vi "Jogo da Velha.vi"(8 "2 Jogadores?":bool=TRUE, 9 "NívelDificuldade":u32, 10 "Jogador 2":string="Jogador 2", 11 "Jogador 1":string="Jogador 1") -> (2 "JogarNovamente?":bool)   [LabVIEW 2011]
doc: "VI responsável por gerenciar o Jogo da Velha, ou seja, a vez de cada jogador, as jogadas feitas e etc."
uses:
  TypeDef/EnumJogadores.ctl
  <vilib>/Utility/sysdir.llb/System Directory Type.ctl
panel:
  in  "JogarNovamente":bool
  out "2x3":string
  in  "stop":bool
  out "Quem joga":string
  out "1x1":string
  out "1x2":string
  out "1x3":string
  out "2x1":string
  out "2x2":string
  out "3x1":string
  out "3x2":string
  out "3x3":string
  # "Jogo da Velha"
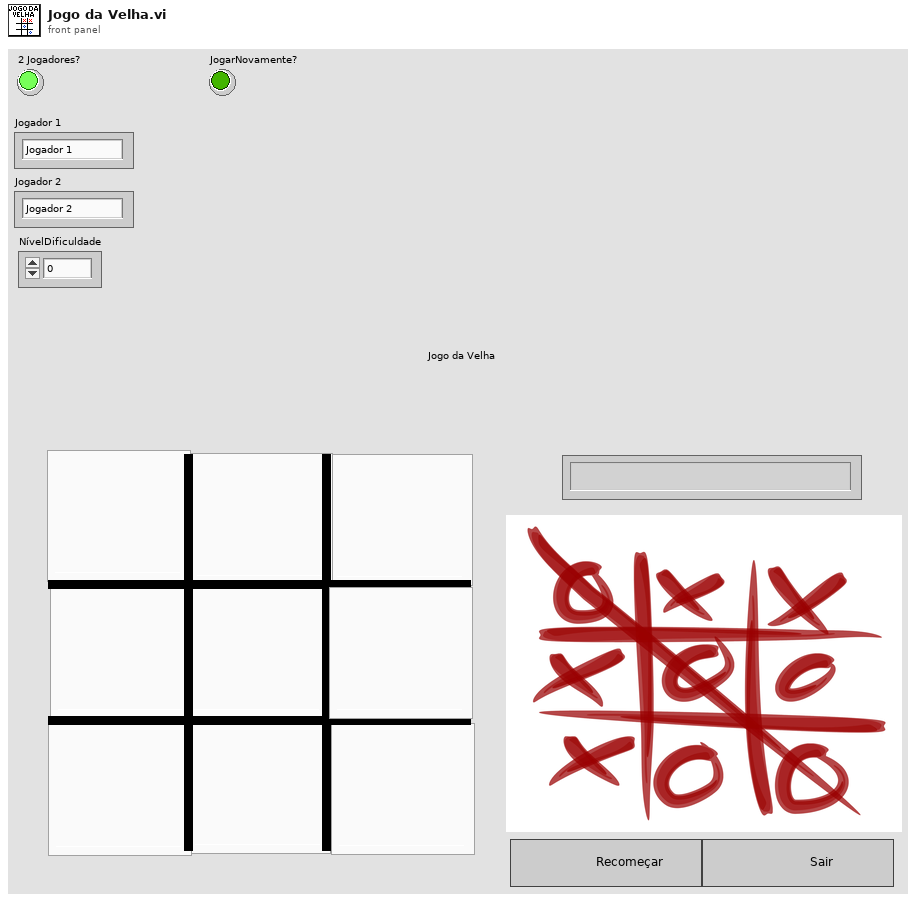
[diagram p1: front panel]
types:
  T1 = typedef "System Directory Type.ctl" = i32
  T2 = enum16{"open", "replace", "create", "open or create", "replace or create", "replace or create with confirmation"}
  T3 = typedef "EnumJogadores.ctl" = enum16{"Jogador 1", "Jogador 2"}
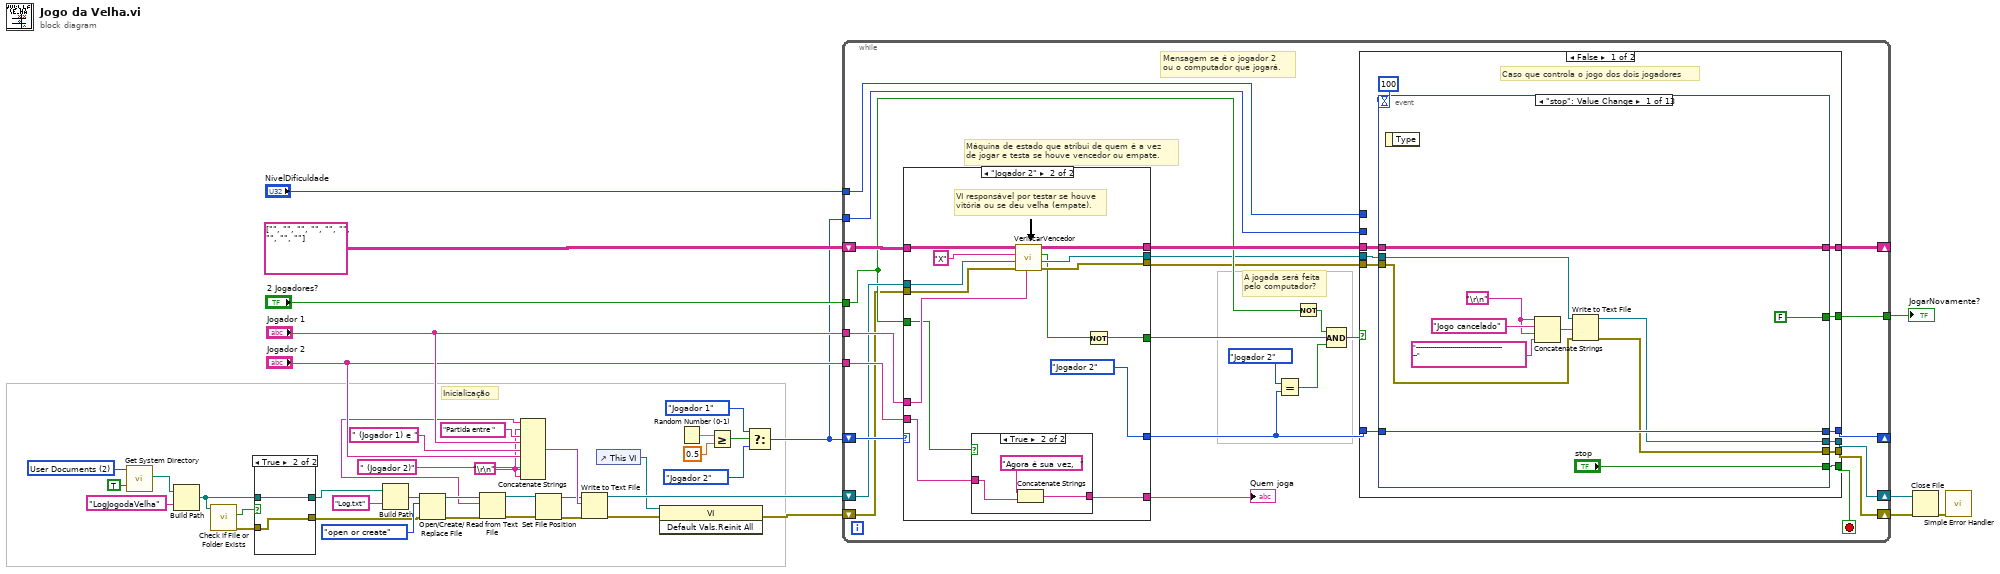
[diagram p0: block diagram]
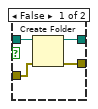
[diagram p2: hidden frame]
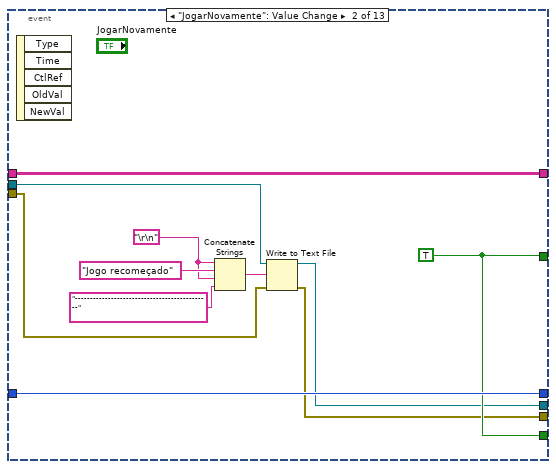
[diagram p3: hidden frame]
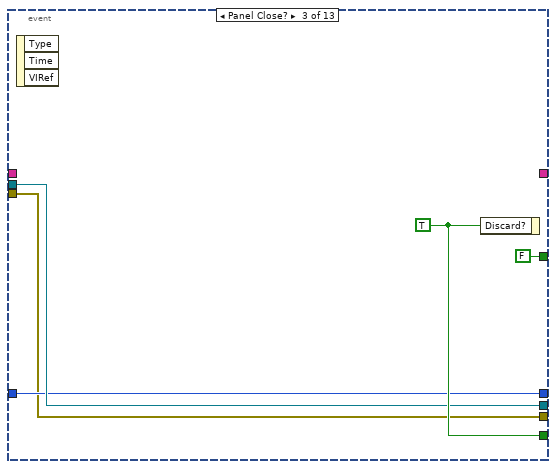
[diagram p4: hidden frame]
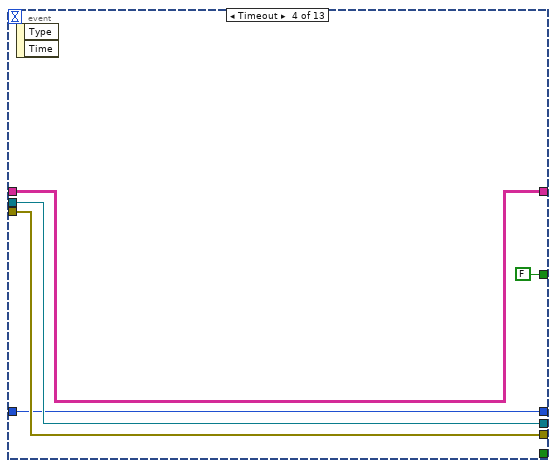
[diagram p5: hidden frame]
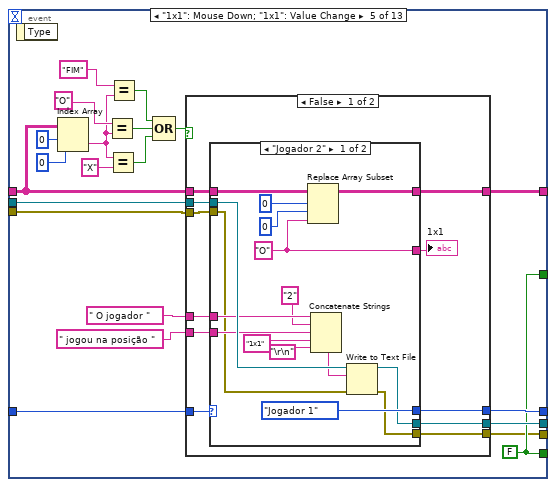
[diagram p6: hidden frame]
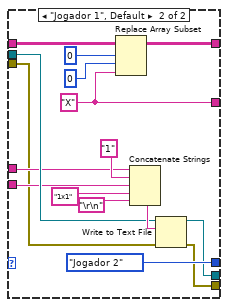
[diagram p7: hidden frame]
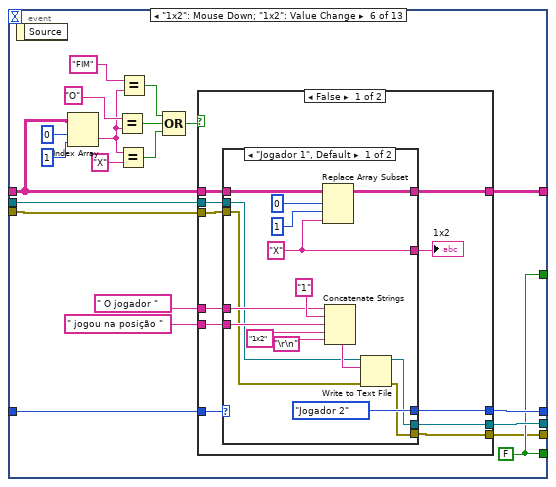
[diagram p9: hidden frame]
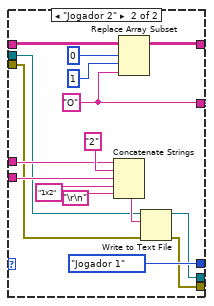
[diagram p10: hidden frame]
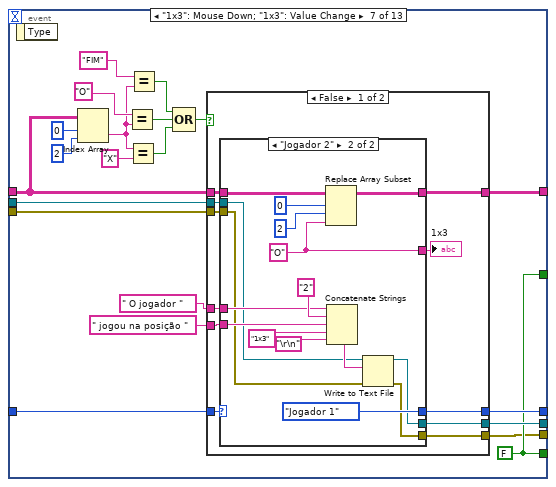
[diagram p12: hidden frame]
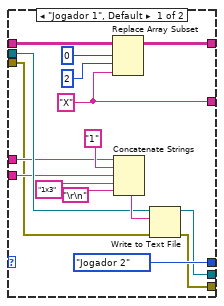
[diagram p13: hidden frame]
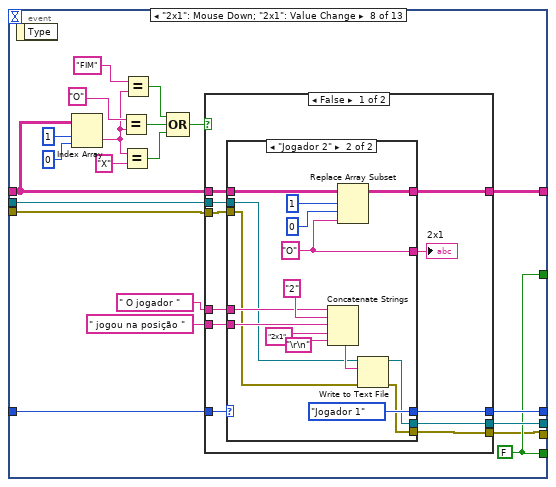
[diagram p15: hidden frame]
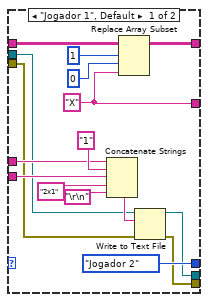
[diagram p16: hidden frame]
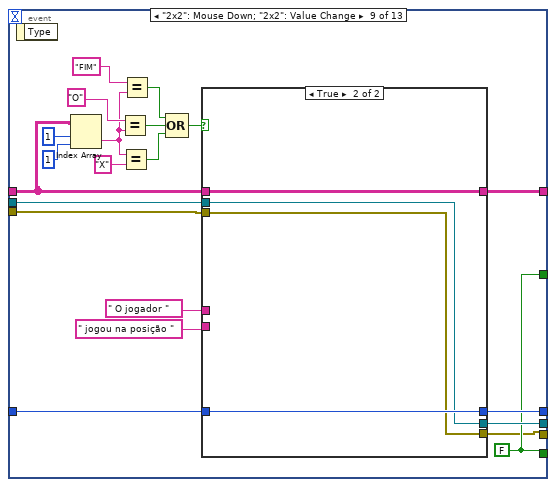
[diagram p18: hidden frame]
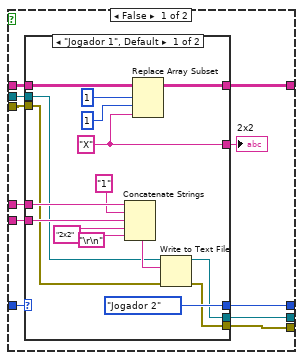
[diagram p19: hidden frame]
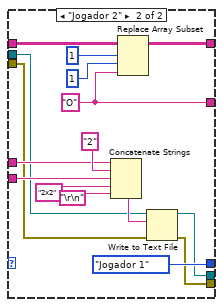
[diagram p20: hidden frame]
diagram:
  w15 = T1 2 items=["User Home"=0, "User Desktop"=1, "User Documents"=2, "User Application Data"=3, "User Preferences"=4, "User Temporary"=5, "Public Documents"=6, "Public Application Data"=7, "Public Preferences"=8, "Public Cache"=13, "System Core Libraries"=9, "System Installed Libraries"=10, "Application Files"=11, "Boot Volume Root"=12] ("system directory type")
  w19 = "\r\n"
  # "Inicialização"
  n1 = call <vilib>:"Get System Directory.vi"("create directory if not found? (F)"=TRUE, "system directory type"=w15) -> ("system directory"=w10:path)  [unwired: 9 in]
  n2 = Build Path(base path=w10, name or relative path="LogJogodaVelha") -> (appended path=w3:path)
  n3 = call <vilib>:"Check if File or Folder Exists.vi"("path"=w3) -> ("error out"=w2:errorcluster, "file or folder exists?"=w1:bool)  [unwired: 8 in, 1 out]
  n4 = case shown="True" w1 {
    tunnel: [w47 w49] -> w8
    tunnel: [w46 w48] -> w7
    tunnel: w3 -> [w45 w49]
    tunnel: w2 -> [w44 w48]
    frame False {
      n5 = Create Folder(path (use dialog)=w45, error in=w44) -> (created path=w47:path, error out=w46:errorcluster)  [unwired: 1 in, 1 out]
    }
    frame True {
    }
  }
  n6 = Build Path(base path=w8, name or relative path="Log.txt") -> (appended path=w13:path)
  n7 = Open/Create/Replace File(file path (use dialog)=w13, error in=w7, operation (0:open)=T2."open or create") -> (refnum out=w27:refnum<file>, error out=w26:errorcluster)  [unwired: 3 in, 1 out]
  n8 = Read from Text File(file (use dialog)=w27, error in=w26) -> (refnum out=w24:refnum<file>, text=w25:string, error out=w22:errorcluster)  [unwired: 2 in, 1 out]
  n9 = Concatenate Strings(w25, w19, "Partida entre " ("string"), "Jogador 1", " (Jogador 1) e " ("string"), "Jogador 2", " (Jogador 2)" ("string"), w19, w19) -> (w31:string)
  n10 = Set File Position(refnum=w24, error in=w22) -> (refnum out=w23:refnum<file>, error out=w21:errorcluster)  [unwired: 2 in]
  n11 = Write to Text File(file (use dialog)=w23, text=w31, error in=w21) -> (refnum out=w29:refnum<file>, error out=w5:errorcluster)  [unwired: 1 in, 1 out]
  n12 = control-ref of="This VI"() -> (w6:refnum<vi>)
  n13 = invoke class="VI" method="Default Vals.Reinit All"(reference=w6, error in=w5) -> (error out=w4:errorcluster)  [unwired: 1 in, 2 out]
  n14 = Random Number (0-1)() -> (number: 0 to 1=w37:dbl)
  n15 = Greater Or Equal?(x=w37, y=0.5) -> (x >= y?=w39:bool)
  n16 = Select(t=EnumJogadores."Jogador 1" ("Enum"), s=w39, f=EnumJogadores."Jogador 2" ("Enum")) -> (s? t:f=w20:T3)
  n17 = while {
    tunnel: "Jogador 2" -> [w70]
    tunnel: "Jogador 1" -> [w71]
    tunnel: "2 Jogadores?" -> [w59]
    shift-right: [w74] -> _
    shift-left: string[][] [["", "", ""], ["", "", ""], ["", "", ""]] ("ArrayJogoVelha") -> [w63]
    shift-right: [w72] -> _
    shift-left: w20 -> [w73]
    tunnel: [w62] -> w36
    shift-right: [w58] -> w28
    shift-left: w29 -> [w60]
    tunnel: w20 -> [w57]
    tunnel: "NívelDificuldade" -> [w51]
    shift-right: [w50] -> w11
    shift-left: w4 -> [w54]
    stop <- w68 stop-if-true
    # "Mensagem se é o jogador 2\nou o computador que jogará."
    # "Máquina de estado que atribui de quem é a vez \nde jogar e testa se houve vencedor ou empate."
    # "A jogada será feita\npelo computador?"
    n18 = case shown="\"Jogador 2\"" w73 {
      tunnel: [EnumJogadores."Jogador 1" ("Enum") EnumJogadores."Jogador 2" ("Enum")] -> w66
      tunnel: w71 -> [w783 w791]
      tunnel: w70 -> [w779 w797]
      tunnel: [w785 w800] -> w69
      tunnel: w59 -> [_ w787]
      tunnel: w63 -> [w784 w798]
      tunnel: [w782 w796] -> w61
      tunnel: w60 -> [w777 w789]
      tunnel: [w780 w794] -> w55
      tunnel: w54 -> [w778 w790]
      tunnel: [w776 w793] -> w53
      tunnel: [w775 w792] -> w52
      frame "Jogador 1" {
        # "VI responsável por testar se houve\nvitória ou se deu velha (empate)."
        n19 = call "VerificarVencedor.vi"("Nome do Jogador"=w779, "error in (no error)"=w778, "refnum in"=w777, "CaracterComparacao"="O", "ArrayEntrada"=w784) -> ("error out"=w775:errorcluster, "refnum out"=w776:refnum<file>, "VenceuOuEmpatou"=w774:bool, "ArraySaida"=w782:string[][])  [unwired: 3 in]
        n20 = Concatenate Strings("Agora é sua vez,  " ("string"), w783) -> (w785:string)
        n21 = Not(x=w774) -> (.not. x?=w780:bool)
      }
      frame "Jogador 2" {
        # "VI responsável por testar se houve\nvitória ou se deu velha (empate)."
        n22 = case shown="True" w787 {
          tunnel: w797 -> [_ w802]
          tunnel: ["Agora é a vez do computador" w803] -> w800
          frame False {
          }
          frame True {
            n23 = Concatenate Strings("Agora é sua vez,  " ("string"), w802) -> (w803:string)
          }
        }
        n24 = call "VerificarVencedor.vi"("Nome do Jogador"=w791, "error in (no error)"=w790, "refnum in"=w789, "CaracterComparacao"="X", "ArrayEntrada"=w798) -> ("error out"=w792:errorcluster, "refnum out"=w793:refnum<file>, "VenceuOuEmpatou"=w788:bool, "ArraySaida"=w796:string[][])  [unwired: 3 in]
        n25 = Not(x=w788) -> (.not. x?=w794:bool)
      }
    }
    "Quem joga" <- w69
    n26 = Equal?(x=EnumJogadores."Jogador 2" ("Enum"), y=w66) -> (x = y?=w56:bool)
    n27 = Not(x=w59) -> (.not. x?=w64:bool)
    n28 = Compound Arithmetic op=AND(w64, w55, w56) -> (w67:bool)
    n29 = case shown="False" w67 {
      tunnel: w61 -> [w85 w732]
      tunnel: [w84 w739] -> w74
      tunnel: w66 -> [w83 _]
      tunnel: [w82 EnumJogadores."Jogador 1" ("Enum")] -> w72
      tunnel: [w81 FALSE ("stop")] -> w68
      tunnel: [w80 FALSE] -> w62
      tunnel: w53 -> [w78 w738]
      tunnel: [w79 w737] -> w58
      tunnel: w57 -> [_ w742]
      tunnel: w52 -> [w77 w734]
      tunnel: [w76 w736] -> w50
      tunnel: w51 -> [_ w735]
      frame False {
        # "Caso que controla o jogo dos dois jogadores"
        n30 = event shown="[0] \"stop\": Value Change" {
          selector: _ -> [_ _ _ _ _ _ _ _ _ _ _ _ _]
          dyn-events: _ -> [_ _ _ _ _ _ _ _ _ _ _ _ _]
          timeout: 100 -> [_ _ _ _ _ _ _ _ _ _ _ _ _]
          tunnel: w85 -> [w96 w108 _ w114 w138 w195 w264 w331 w400 w467 w536 w604 w672]
          tunnel: [w96 w108 _ w114 w139 w207 w275 w343 w411 w479 w547 w615 w683] -> w84
          tunnel: w83 -> [w95 w107 w111 w115 w135 w206 w274 w342 w410 w478 w546 w614 w682]
          tunnel: [w95 w107 w111 w115 w134 w205 w273 w341 w409 w477 w545 w613 w681] -> w82
          tunnel: ["stop" w106 w113 _ w121 w190 w257 w325 w393 w461 w529 w597 w665] -> w81
          tunnel: [FALSE w106 FALSE FALSE w121 w190 w257 w325 w393 w461 w529 w597 w665] -> w80
          tunnel: w78 -> [w90 w102 w112 w118 w125 w189 w261 w329 w397 w465 w533 w601 w669]
          tunnel: [w89 w101 w112 w118 w124 w193 w260 w328 w396 w464 w532 w600 w668] -> w79
          tunnel: w77 -> [w87 w99 w110 w117 w120 w188 w256 w324 w392 w460 w528 w596 w664]
          tunnel: [w86 w98 w110 w117 w119 w187 w255 w323 w391 w459 w527 w595 w663] -> w76
          event "stop": Value Change {
            w91 = "\r\n"
            n31 = event-data() -> ()  [unwired: 1 in, 1 out]
            n32 = Concatenate Strings(w91, "Jogo cancelado" ("string"), w91, "---------------------------------------------" ("string")) -> (w93:string)
            n33 = Write to Text File(file (use dialog)=w90, text=w93, error in=w87) -> (refnum out=w89:refnum<file>, error out=w86:errorcluster)  [unwired: 1 in, 1 out]
          }
          event "JogarNovamente": Value Change {
            w103 = "\r\n"
            w106 = TRUE
            n34 = event-data() -> ()  [unwired: 1 in, 5 out]
            n35 = Concatenate Strings(w103, "Jogo recomeçado" ("string"), w103, "---------------------------------------------" ("string")) -> (w105:string)
            n36 = Write to Text File(file (use dialog)=w102, text=w105, error in=w99) -> (refnum out=w101:refnum<file>, error out=w98:errorcluster)  [unwired: 1 in, 1 out]
          }
          event Panel Close? {
            w113 = TRUE ("Discard?")
            n37 = event-data() -> ()  [unwired: 1 in, 3 out]
            n38 = event-data("Discard?"=w113) -> ()  [unwired: 1 in, 1 out]
          }
          event Timeout {
            n39 = event-data() -> ()  [unwired: 1 in, 2 out]
          }
          event "1x1": Mouse Down; "1x1": Value Change {
            w121 = FALSE
            n40 = event-data() -> ()  [unwired: 1 in, 1 out]
            n41 = Index Array(array=w138, index (row)=0, index (col)=0 ("disabled index (col)")) -> (element=w128:string)
            n42 = Equal?(x="O", y=w128) -> (x = y?=w130:bool)
            n43 = Equal?(x=w128, y="X") -> (x = y?=w131:bool)
            n44 = Equal?(x="FIM", y=w128) -> (x = y?=w126:bool)
            n45 = Compound Arithmetic op=OR(w126, w130, w131) -> (w132:bool)
            n46 = case shown="False" w132 {
              tunnel: w138 -> [w150 w186]
              tunnel: [w149 w186] -> w139
              tunnel: w135 -> [w147 w183]
              tunnel: [w146 w183] -> w134
              tunnel: w125 -> [w145 w185]
              tunnel: [w144 w185] -> w124
              tunnel: " O jogador " ("string") -> [w143 _]
              tunnel: " jogou na posição " ("string") -> [w142 _]
              tunnel: w120 -> [w141 w184]
              tunnel: [w140 w184] -> w119
              frame False {
                n47 = case shown="\"Jogador 2\"" w147 {
                  tunnel: w150 -> [w164 w180]
                  tunnel: [w163 w179] -> w149
                  tunnel: [w162 w178] -> w148
                  tunnel: [EnumJogadores."Jogador 1" ("Enum") EnumJogadores."Jogador 2" ("Enum")] -> w146
                  tunnel: w145 -> [w159 w172]
                  tunnel: [w160 w169] -> w144
                  tunnel: w143 -> [w157 w171]
                  tunnel: w142 -> [w156 w170]
                  tunnel: w141 -> [w152 w168]
                  tunnel: [w151 w167] -> w140
                  frame "Jogador 2" {
                    w162 = "O" ("new element/subarray")
                    n48 = Replace Array Subset(array=w164, new element=w162, index (row)=0, index (col)=0 ("disabled index (col)")) -> (w163:string[][])
                    n49 = Concatenate Strings(w157, "2" ("string"), w156, "1x1" ("string"), "\r\n") -> (w158:string)
                    n50 = Write to Text File(file (use dialog)=w159, text=w158, error in=w152) -> (refnum out=w160:refnum<file>, error out=w151:errorcluster)  [unwired: 1 in, 1 out]
                  }
                  frame "Jogador 1", Default {
                    w178 = "X" ("new element/subarray")
                    n51 = Replace Array Subset(array=w180, new element=w178, index (row)=0, index (col)=0 ("disabled index (col)")) -> (w179:string[][])
                    n52 = Concatenate Strings(w171, "1" ("string"), w170, "1x1" ("string"), "\r\n") -> (w173:string)
                    n53 = Write to Text File(file (use dialog)=w172, text=w173, error in=w168) -> (refnum out=w169:refnum<file>, error out=w167:errorcluster)  [unwired: 1 in, 1 out]
                  }
                }
                "1x1" <- w148
              }
              frame True {
              }
            }
          }
          event "1x2": Mouse Down; "1x2": Value Change {
            w190 = FALSE
            n54 = event-data() -> ()  [unwired: 1 in, 1 out]
            n55 = Index Array(array=w195, index (row)=0, index (col)=1 ("disabled index (col)")) -> (element=w200:string)
            n56 = Equal?(x="O", y=w200) -> (x = y?=w202:bool)
            n57 = Equal?(x=w200, y="X") -> (x = y?=w203:bool)
            n58 = Equal?(x="FIM", y=w200) -> (x = y?=w198:bool)
            n59 = Compound Arithmetic op=OR(w198, w202, w203) -> (w194:bool)
            n60 = case shown="False" w194 {
              tunnel: w195 -> [w218 w254]
              tunnel: [w217 w254] -> w207
              tunnel: w206 -> [w215 w253]
              tunnel: [w214 w253] -> w205
              tunnel: w189 -> [w213 w252]
              tunnel: [w212 w252] -> w193
              tunnel: " O jogador " ("string") -> [w211 _]
              tunnel: " jogou na posição " ("string") -> [w210 _]
              tunnel: w188 -> [w209 w251]
              tunnel: [w208 w251] -> w187
              frame False {
                n61 = case shown="\"Jogador 1\", Default" w215 {
                  tunnel: w218 -> [w234 w248]
                  tunnel: [w233 w247] -> w217
                  tunnel: [w230 w246] -> w216
                  tunnel: [EnumJogadores."Jogador 2" ("Enum") EnumJogadores."Jogador 1" ("Enum")] -> w214
                  tunnel: w213 -> [w221 w237]
                  tunnel: [w222 w238] -> w212
                  tunnel: w211 -> [w224 w240]
                  tunnel: w210 -> [w223 w239]
                  tunnel: w209 -> [w220 w236]
                  tunnel: [w219 w235] -> w208
                  frame "Jogador 1", Default {
                    w230 = "X" ("new element/subarray")
                    n62 = Replace Array Subset(array=w234, new element=w230, index (row)=0, index (col)=1 ("disabled index (col)")) -> (w233:string[][])
                    n63 = Concatenate Strings(w224, "1" ("string"), w223, "1x2" ("string"), "\r\n") -> (w225:string)
                    n64 = Write to Text File(file (use dialog)=w221, text=w225, error in=w220) -> (refnum out=w222:refnum<file>, error out=w219:errorcluster)  [unwired: 1 in, 1 out]
                  }
                  frame "Jogador 2" {
                    w246 = "O" ("new element/subarray")
                    n65 = Concatenate Strings(w240, "2" ("string"), w239, "1x2" ("string"), "\r\n") -> (w241:string)
                    n66 = Replace Array Subset(array=w248, new element=w246, index (row)=0, index (col)=1 ("disabled index (col)")) -> (w247:string[][])
                    n67 = Write to Text File(file (use dialog)=w237, text=w241, error in=w236) -> (refnum out=w238:refnum<file>, error out=w235:errorcluster)  [unwired: 1 in, 1 out]
                  }
                }
                "1x2" <- w216
              }
              frame True {
              }
            }
          }
          event "1x3": Mouse Down; "1x3": Value Change {
            w257 = FALSE
            n68 = event-data() -> ()  [unwired: 1 in, 1 out]
            n69 = Index Array(array=w264, index (row)=0, index (col)=2 ("disabled index (col)")) -> (element=w268:string)
            n70 = Equal?(x="O", y=w268) -> (x = y?=w270:bool)
            n71 = Equal?(x=w268, y="X") -> (x = y?=w271:bool)
            n72 = Equal?(x="FIM", y=w268) -> (x = y?=w266:bool)
            n73 = Compound Arithmetic op=OR(w266, w270, w271) -> (w263:bool)
            n74 = case shown="False" w263 {
              tunnel: w264 -> [w286 w322]
              tunnel: [w285 w322] -> w275
              tunnel: w274 -> [w283 w321]
              tunnel: [w282 w321] -> w273
              tunnel: w261 -> [w281 w320]
              tunnel: [w280 w320] -> w260
              tunnel: " jogou na posição " ("string") -> [w279 _]
              tunnel: " O jogador " ("string") -> [w278 _]
              tunnel: w256 -> [w277 w319]
              tunnel: [w276 w319] -> w255
              frame False {
                n75 = case shown="\"Jogador 2\"" w283 {
                  tunnel: w286 -> [w300 w316]
                  tunnel: [w299 w315] -> w285
                  tunnel: [w298 w314] -> w284
                  tunnel: [EnumJogadores."Jogador 2" ("Enum") EnumJogadores."Jogador 1" ("Enum")] -> w282
                  tunnel: w281 -> [w291 w305]
                  tunnel: [w292 w306] -> w280
                  tunnel: w279 -> [w289 w307]
                  tunnel: w278 -> [w290 w308]
                  tunnel: w277 -> [w288 w304]
                  tunnel: [w287 w303] -> w276
                  frame "Jogador 1", Default {
                    w298 = "X" ("new element/subarray")
                    n76 = Replace Array Subset(array=w300, new element=w298, index (row)=0, index (col)=2 ("disabled index (col)")) -> (w299:string[][])
                    n77 = Concatenate Strings(w290, "1" ("string"), w289, "1x3" ("string"), "\r\n") -> (w296:string)
                    n78 = Write to Text File(file (use dialog)=w291, text=w296, error in=w288) -> (refnum out=w292:refnum<file>, error out=w287:errorcluster)  [unwired: 1 in, 1 out]
                  }
                  frame "Jogador 2" {
                    w314 = "O" ("new element/subarray")
                    n79 = Replace Array Subset(array=w316, new element=w314, index (row)=0, index (col)=2 ("disabled index (col)")) -> (w315:string[][])
                    n80 = Concatenate Strings(w308, "2" ("string"), w307, "1x3" ("string"), "\r\n") -> (w309:string)
                    n81 = Write to Text File(file (use dialog)=w305, text=w309, error in=w304) -> (refnum out=w306:refnum<file>, error out=w303:errorcluster)  [unwired: 1 in, 1 out]
                  }
                }
                "1x3" <- w284
              }
              frame True {
              }
            }
          }
          event "2x1": Mouse Down; "2x1": Value Change {
            w325 = FALSE
            n82 = event-data() -> ()  [unwired: 1 in, 1 out]
            n83 = Index Array(array=w331, index (row)=1, index (col)=0 ("disabled index (col)")) -> (element=w336:string)
            n84 = Equal?(x="O", y=w336) -> (x = y?=w338:bool)
            n85 = Equal?(x=w336, y="X") -> (x = y?=w339:bool)
            n86 = Equal?(x="FIM", y=w336) -> (x = y?=w334:bool)
            n87 = Compound Arithmetic op=OR(w334, w338, w339) -> (w330:bool)
            n88 = case shown="False" w330 {
              tunnel: w331 -> [w354 w390]
              tunnel: [w353 w390] -> w343
              tunnel: w342 -> [w351 w389]
              tunnel: [w350 w389] -> w341
              tunnel: w329 -> [w349 w387]
              tunnel: [w348 w387] -> w328
              tunnel: " O jogador " ("string") -> [w347 _]
              tunnel: " jogou na posição " ("string") -> [w346 _]
              tunnel: w324 -> [w345 w388]
              tunnel: [w344 w388] -> w323
              frame False {
                n89 = case shown="\"Jogador 2\"" w351 {
                  tunnel: w354 -> [w368 w384]
                  tunnel: [w367 w383] -> w353
                  tunnel: [w366 w382] -> w352
                  tunnel: [EnumJogadores."Jogador 2" ("Enum") EnumJogadores."Jogador 1" ("Enum")] -> w350
                  tunnel: w349 -> [w357 w373]
                  tunnel: [w358 w376] -> w348
                  tunnel: w347 -> [w360 w375]
                  tunnel: w346 -> [w359 w374]
                  tunnel: w345 -> [w356 w372]
                  tunnel: [w355 w371] -> w344
                  frame "Jogador 1", Default {
                    w366 = "X" ("new element/subarray")
                    n90 = Concatenate Strings(w360, "1" ("string"), w359, "2x1" ("string"), "\r\n") -> (w361:string)
                    n91 = Replace Array Subset(array=w368, new element=w366, index (row)=1, index (col)=0 ("disabled index (col)")) -> (w367:string[][])
                    n92 = Write to Text File(file (use dialog)=w357, text=w361, error in=w356) -> (refnum out=w358:refnum<file>, error out=w355:errorcluster)  [unwired: 1 in, 1 out]
                  }
                  frame "Jogador 2" {
                    w382 = "O" ("new element/subarray")
                    n93 = Concatenate Strings(w375, "2" ("string"), w374, "2x1" ("string"), "\r\n") -> (w378:string)
                    n94 = Replace Array Subset(array=w384, new element=w382, index (row)=1, index (col)=0 ("disabled index (col)")) -> (w383:string[][])
                    n95 = Write to Text File(file (use dialog)=w373, text=w378, error in=w372) -> (refnum out=w376:refnum<file>, error out=w371:errorcluster)  [unwired: 1 in, 1 out]
                  }
                }
                "2x1" <- w352
              }
              frame True {
              }
            }
          }
          event "2x2": Mouse Down; "2x2": Value Change {
            w393 = FALSE
            n96 = event-data() -> ()  [unwired: 1 in, 1 out]
            n97 = Index Array(array=w400, index (row)=1, index (col)=1 ("disabled index (col)")) -> (element=w404:string)
            n98 = Equal?(x="O", y=w404) -> (x = y?=w406:bool)
            n99 = Equal?(x=w404, y="X") -> (x = y?=w407:bool)
            n100 = Equal?(x="FIM", y=w404) -> (x = y?=w402:bool)
            n101 = Compound Arithmetic op=OR(w402, w406, w407) -> (w398:bool)
            n102 = case shown="True" w398 {
              tunnel: w400 -> [w422 w458]
              tunnel: [w421 w458] -> w411
              tunnel: w410 -> [w419 w457]
              tunnel: [w418 w457] -> w409
              tunnel: w397 -> [w417 w456]
              tunnel: [w414 w456] -> w396
              tunnel: " O jogador " ("string") -> [w416 _]
              tunnel: " jogou na posição " ("string") -> [w415 _]
              tunnel: w392 -> [w413 w455]
              tunnel: [w412 w455] -> w391
              frame False {
                n103 = case shown="\"Jogador 1\", Default" w419 {
                  tunnel: w422 -> [w436 w452]
                  tunnel: [w435 w451] -> w421
                  tunnel: [w434 w450] -> w420
                  tunnel: [EnumJogadores."Jogador 2" ("Enum") EnumJogadores."Jogador 1" ("Enum")] -> w418
                  tunnel: w417 -> [w425 w441]
                  tunnel: w416 -> [w429 w444]
                  tunnel: w415 -> [w428 w443]
                  tunnel: [w426 w442] -> w414
                  tunnel: w413 -> [w424 w440]
                  tunnel: [w423 w439] -> w412
                  frame "Jogador 1", Default {
                    w434 = "X" ("new element/subarray")
                    n104 = Concatenate Strings(w429, "1" ("string"), w428, "2x2" ("string"), "\r\n") -> (w430:string)
                    n105 = Replace Array Subset(array=w436, new element=w434, index (row)=1, index (col)=1 ("disabled index (col)")) -> (w435:string[][])
                    n106 = Write to Text File(file (use dialog)=w425, text=w430, error in=w424) -> (refnum out=w426:refnum<file>, error out=w423:errorcluster)  [unwired: 1 in, 1 out]
                  }
                  frame "Jogador 2" {
                    w450 = "O" ("new element/subarray")
                    n107 = Concatenate Strings(w444, "2" ("string"), w443, "2x2" ("string"), "\r\n") -> (w446:string)
                    n108 = Replace Array Subset(array=w452, new element=w450, index (row)=1, index (col)=1 ("disabled index (col)")) -> (w451:string[][])
                    n109 = Write to Text File(file (use dialog)=w441, text=w446, error in=w440) -> (refnum out=w442:refnum<file>, error out=w439:errorcluster)  [unwired: 1 in, 1 out]
                  }
                }
                "2x2" <- w420
              }
              frame True {
              }
            }
          }
          event "2x3": Mouse Down; "2x3": Value Change {
            w461 = FALSE
            n110 = event-data() -> ()  [unwired: 1 in, 1 out]
            n111 = Index Array(array=w467, index (row)=1, index (col)=2 ("disabled index (col)")) -> (element=w472:string)
            n112 = Equal?(x="O", y=w472) -> (x = y?=w474:bool)
            n113 = Equal?(x=w472, y="X") -> (x = y?=w475:bool)
            n114 = Equal?(x="FIM", y=w472) -> (x = y?=w470:bool)
            n115 = Compound Arithmetic op=OR(w470, w474, w475) -> (w466:bool)
            n116 = case shown="True" w466 {
              tunnel: w467 -> [w490 w526]
              tunnel: [w489 w526] -> w479
              tunnel: w478 -> [w484 w525]
              tunnel: [w487 w525] -> w477
              tunnel: w465 -> [w486 w524]
              tunnel: [w485 w524] -> w464
              tunnel: " O jogador " ("string") -> [w483 _]
              tunnel: " jogou na posição " ("string") -> [w482 _]
              tunnel: w460 -> [w481 w523]
              tunnel: [w480 w523] -> w459
              frame False {
                n117 = case shown="\"Jogador 2\"" w484 {
                  tunnel: w490 -> [w504 w521]
                  tunnel: [w503 w520] -> w489
                  tunnel: [w502 w518] -> w488
                  tunnel: [EnumJogadores."Jogador 2" ("Enum") EnumJogadores."Jogador 1" ("Enum")] -> w487
                  tunnel: w486 -> [w494 w512]
                  tunnel: [w493 w511] -> w485
                  tunnel: w483 -> [w496 w510]
                  tunnel: w482 -> [w495 w509]
                  tunnel: w481 -> [w492 w508]
                  tunnel: [w491 w507] -> w480
                  frame "Jogador 1", Default {
                    w502 = "X" ("new element/subarray")
                    n118 = Concatenate Strings(w496, "1" ("string"), w495, "2x3" ("string"), "\r\n") -> (w497:string)
                    n119 = Replace Array Subset(array=w504, new element=w502, index (row)=1, index (col)=2 ("disabled index (col)")) -> (w503:string[][])
                    n120 = Write to Text File(file (use dialog)=w494, text=w497, error in=w492) -> (refnum out=w493:refnum<file>, error out=w491:errorcluster)  [unwired: 1 in, 1 out]
                  }
                  frame "Jogador 2" {
                    w518 = "O" ("new element/subarray")
                    n121 = Concatenate Strings(w510, "2" ("string"), w509, "2x3" ("string"), "\r\n") -> (w513:string)
                    n122 = Replace Array Subset(array=w521, new element=w518, index (row)=1, index (col)=2 ("disabled index (col)")) -> (w520:string[][])
                    n123 = Write to Text File(file (use dialog)=w512, text=w513, error in=w508) -> (refnum out=w511:refnum<file>, error out=w507:errorcluster)  [unwired: 1 in, 1 out]
                  }
                }
                "2x3" <- w488
              }
              frame True {
              }
            }
          }
          event "3x1": Mouse Down; "3x1": Value Change {
            w529 = FALSE
            n124 = event-data() -> ()  [unwired: 1 in, 1 out]
            n125 = Index Array(array=w536, index (row)=2, index (col)=0 ("disabled index (col)")) -> (element=w540:string)
            n126 = Equal?(x="O", y=w540) -> (x = y?=w542:bool)
            n127 = Equal?(x=w540, y="X") -> (x = y?=w543:bool)
            n128 = Equal?(x="FIM", y=w540) -> (x = y?=w538:bool)
            n129 = Compound Arithmetic op=OR(w538, w542, w543) -> (w537:bool)
            n130 = case shown="False" w537 {
              tunnel: w536 -> [w558 w594]
              tunnel: [w557 w594] -> w547
              tunnel: w546 -> [w555 w593]
              tunnel: [w554 w593] -> w545
              tunnel: w533 -> [w553 w592]
              tunnel: [w552 w592] -> w532
              tunnel: " O jogador " ("string") -> [w551 _]
              tunnel: " jogou na posição " ("string") -> [w550 _]
              tunnel: w528 -> [w549 w591]
              tunnel: [w548 w591] -> w527
              frame False {
                n131 = case shown="\"Jogador 2\"" w555 {
                  tunnel: w558 -> [w572 w588]
                  tunnel: [w571 w587] -> w557
                  tunnel: [w570 w586] -> w556
                  tunnel: [EnumJogadores."Jogador 2" ("Enum") EnumJogadores."Jogador 1" ("Enum")] -> w554
                  tunnel: w553 -> [w561 w577]
                  tunnel: [w562 w580] -> w552
                  tunnel: w551 -> [w564 w579]
                  tunnel: w550 -> [w563 w578]
                  tunnel: w549 -> [w560 w576]
                  tunnel: [w559 w575] -> w548
                  frame "Jogador 1", Default {
                    w570 = "X" ("new element/subarray")
                    n132 = Concatenate Strings(w564, "1" ("string"), w563, "3x1" ("string"), "\r\n") -> (w565:string)
                    n133 = Replace Array Subset(array=w572, new element=w570, index (row)=2, index (col)=0 ("disabled index (col)")) -> (w571:string[][])
                    n134 = Write to Text File(file (use dialog)=w561, text=w565, error in=w560) -> (refnum out=w562:refnum<file>, error out=w559:errorcluster)  [unwired: 1 in, 1 out]
                  }
                  frame "Jogador 2" {
                    w586 = "O" ("new element/subarray")
                    n135 = Concatenate Strings(w579, "2" ("string"), w578, "3x1" ("string"), "\r\n") -> (w581:string)
                    n136 = Replace Array Subset(array=w588, new element=w586, index (row)=2, index (col)=0 ("disabled index (col)")) -> (w587:string[][])
                    n137 = Write to Text File(file (use dialog)=w577, text=w581, error in=w576) -> (refnum out=w580:refnum<file>, error out=w575:errorcluster)  [unwired: 1 in, 1 out]
                  }
                }
                "3x1" <- w556
              }
              frame True {
              }
            }
          }
          event "3x2": Mouse Down; "3x2": Value Change {
            w597 = FALSE
            n138 = event-data() -> ()  [unwired: 1 in, 1 out]
            n139 = Index Array(array=w604, index (row)=2, index (col)=1 ("disabled index (col)")) -> (element=w608:string)
            n140 = Equal?(x="O", y=w608) -> (x = y?=w610:bool)
            n141 = Equal?(x=w608, y="X") -> (x = y?=w611:bool)
            n142 = Equal?(x="FIM", y=w608) -> (x = y?=w606:bool)
            n143 = Compound Arithmetic op=OR(w606, w610, w611) -> (w602:bool)
            n144 = case shown="False" w602 {
              tunnel: [w626 w662] -> w615
              tunnel: w614 -> [w623 w661]
              tunnel: w604 -> [w624 w662]
              tunnel: [w622 w661] -> w613
              tunnel: w601 -> [w621 w660]
              tunnel: [w620 w660] -> w600
              tunnel: " O jogador " ("string") -> [w619 _]
              tunnel: " jogou na posição " ("string") -> [w618 _]
              tunnel: w596 -> [w617 w659]
              tunnel: [w616 w659] -> w595
              frame False {
                n145 = case shown="\"Jogador 2\"" w623 {
                  tunnel: w624 -> [w640 w656]
                  tunnel: [w639 w654] -> w626
                  tunnel: [w638 w655] -> w625
                  tunnel: [EnumJogadores."Jogador 2" ("Enum") EnumJogadores."Jogador 1" ("Enum")] -> w622
                  tunnel: w621 -> [w629 w645]
                  tunnel: [w632 w646] -> w620
                  tunnel: w619 -> [w631 w648]
                  tunnel: w618 -> [w630 w647]
                  tunnel: w617 -> [w628 w644]
                  tunnel: [w627 w643] -> w616
                  frame "Jogador 1", Default {
                    w638 = "X" ("new element/subarray")
                    n146 = Concatenate Strings(w631, "1" ("string"), w630, "3x2" ("string"), "\r\n") -> (w633:string)
                    n147 = Replace Array Subset(array=w640, new element=w638, index (row)=2, index (col)=1 ("disabled index (col)")) -> (w639:string[][])
                    n148 = Write to Text File(file (use dialog)=w629, text=w633, error in=w628) -> (refnum out=w632:refnum<file>, error out=w627:errorcluster)  [unwired: 1 in, 1 out]
                  }
                  frame "Jogador 2" {
                    w655 = "O" ("new element/subarray")
                    n149 = Concatenate Strings(w648, "2" ("string"), w647, "3x2" ("string"), "\r\n") -> (w649:string)
                    n150 = Replace Array Subset(array=w656, new element=w655, index (row)=2, index (col)=1 ("disabled index (col)")) -> (w654:string[][])
                    n151 = Write to Text File(file (use dialog)=w645, text=w649, error in=w644) -> (refnum out=w646:refnum<file>, error out=w643:errorcluster)  [unwired: 1 in, 1 out]
                  }
                }
                "3x2" <- w625
              }
              frame True {
              }
            }
          }
          event "3x3": Mouse Down; "3x3": Value Change {
            w665 = FALSE
            n152 = event-data() -> ()  [unwired: 1 in, 1 out]
            n153 = Index Array(array=w672, index (row)=2, index (col)=2 ("disabled index (col)")) -> (element=w676:string)
            n154 = Equal?(x="O", y=w676) -> (x = y?=w678:bool)
            n155 = Equal?(x=w676, y="X") -> (x = y?=w679:bool)
            n156 = Equal?(x="FIM", y=w676) -> (x = y?=w674:bool)
            n157 = Compound Arithmetic op=OR(w674, w678, w679) -> (w670:bool)
            n158 = case shown="False" w670 {
              tunnel: w672 -> [w694 w730]
              tunnel: [w693 w730] -> w683
              tunnel: w682 -> [w691 w729]
              tunnel: [w690 w729] -> w681
              tunnel: w669 -> [w689 w728]
              tunnel: [w688 w728] -> w668
              tunnel: " O jogador " ("string") -> [w687 _]
              tunnel: " jogou na posição " ("string") -> [w686 _]
              tunnel: w664 -> [w685 w727]
              tunnel: [w684 w727] -> w663
              frame False {
                n159 = case shown="\"Jogador 1\", Default" w691 {
                  tunnel: w694 -> [w708 w724]
                  tunnel: [w707 w723] -> w693
                  tunnel: [w706 w722] -> w692
                  tunnel: [EnumJogadores."Jogador 2" ("Enum") EnumJogadores."Jogador 1" ("Enum")] -> w690
                  tunnel: w689 -> [w697 w713]
                  tunnel: [w700 w716] -> w688
                  tunnel: w687 -> [w698 w715]
                  tunnel: w686 -> [w699 w714]
                  tunnel: w685 -> [w696 w712]
                  tunnel: [w695 w711] -> w684
                  frame "Jogador 1", Default {
                    w706 = "X" ("new element/subarray")
                    n160 = Concatenate Strings(w698, "1" ("string"), w699, "3x3" ("string"), "\r\n") -> (w701:string)
                    n161 = Replace Array Subset(array=w708, new element=w706, index (row)=2, index (col)=2 ("disabled index (col)")) -> (w707:string[][])
                    n162 = Write to Text File(file (use dialog)=w697, text=w701, error in=w696) -> (refnum out=w700:refnum<file>, error out=w695:errorcluster)  [unwired: 1 in, 1 out]
                  }
                  frame "Jogador 2" {
                    w722 = "O" ("new element/subarray")
                    n163 = Concatenate Strings(w715, "2" ("string"), w714, "3x3" ("string"), "\r\n") -> (w717:string)
                    n164 = Replace Array Subset(array=w724, new element=w722, index (row)=2, index (col)=2 ("disabled index (col)")) -> (w723:string[][])
                    n165 = Write to Text File(file (use dialog)=w713, text=w717, error in=w712) -> (refnum out=w716:refnum<file>, error out=w711:errorcluster)  [unwired: 1 in, 1 out]
                  }
                }
                "3x3" <- w692
              }
              frame True {
              }
            }
          }
        }
      }
      frame True {
        # "O case abaixo evita que mesmo com o \njogo já terminado seja feita alguma \njogada pela máquina."
        # "Caso que controla o jogo do computador"
        n166 = Equal?(x=string[][] [["FIM", "FIM", "FIM"], ["FIM", "FIM", "FIM"], ["FIM", "FIM", "FIM"]] ("y"), y=w732) -> (x = y?=w733:bool)
        n167 = case shown="False" w733 {
          tunnel: w742 -> [w760 _]
          tunnel: w732 -> [w759 w772]
          tunnel: [w757 w772] -> w739
          tunnel: w738 -> [w754 w770]
          tunnel: [w753 w770] -> w737
          tunnel: [w751 w771] -> w736
          tunnel: w735 -> [w750 _]
          tunnel: w734 -> [w747 w771]
          frame False {
            # "Espera um tempo entre\no limite superior e o\nlimite inferior"
            # "VI resposável por\nfazer as jogadas \ndo computador."
            n168 = call "TempodeEspera.vi"("error in (no error)"=w747, "Limite Inferior (ms)"=200.0, "Limite Superior (ms)"=2000.0) -> ("error out"=w745:errorcluster)  [unwired: 8 in]
            n169 = call "Computador.vi"("Nível de Dificuldade"=w750, "error in (no error)"=w745, "JogodaVelhaIn"=w759, "QuemComecou"=w760) -> ("error out"=w744:errorcluster, "Jogada"=w746:string, "JogadaVelhaOut"=w757:string[][])  [unwired: 5 in]
            n170 = case shown="\"2x0\"" w746 {
              tunnel: "O" ("1x1") -> [w761 w762 w763 w764 w765 w766 w767 w768 _ w769]
              frame "0x1" {
                n171 = local write "1x2"(w761) -> ()
              }
              frame "0x2" {
                n172 = local write "1x3"(w762) -> ()
              }
              frame "1x0" {
                n173 = local write "2x1"(w763) -> ()
              }
              frame "1x1" {
                n174 = local write "2x2"(w764) -> ()
              }
              frame "1x2" {
                n175 = local write "2x3"(w765) -> ()
              }
              frame "2x0" {
                n176 = local write "3x1"(w766) -> ()
              }
              frame "2x1" {
                n177 = local write "3x2"(w767) -> ()
              }
              frame "2x2" {
                n178 = local write "3x3"(w768) -> ()
              }
              frame "Nada", Default {
              }
              frame "0x0" {
                n179 = local write "1x1"(w769) -> ()
              }
            }
            n180 = Concatenate Strings("O computador jogou na posição ", w746, "\r\n") -> (w756:string)
            n181 = Write to Text File(file (use dialog)=w754, text=w756, error in=w744) -> (refnum out=w753:refnum<file>, error out=w751:errorcluster)  [unwired: 1 in, 1 out]
          }
          frame True {
          }
        }
      }
    }
  }
  "JogarNovamente?" <- w36
  n182 = Close File(refnum=w28, error in=w11) -> (error out=w17:errorcluster)  [unwired: 1 out]
  n183 = call <vilib>:"Simple Error Handler.vi"("error in (no error)"=w17) -> ()  [unwired: 4 in, 5 out]
